vi "Write Record.vi"(8 "error in (no error)":errorcluster, 10 "Record":T1 {"Balance" format="%_4p"}, 11 "Simulated Configuration Database Actor in":refnum<class "Configuration Database Actor.lvclass">) -> (0 "error out":errorcluster, 3 "Simulated Configuration Database Actor out":refnum<class "Configuration Database Actor.lvclass">)   [LabVIEW 2019, in "Configuration Database Actor.lvlib" / "Configuration Database Actor.lvclass"]
uses:
  Configuration Database Actor.lvclass
  Records -cluster.ctl
  Configuration Database Actor.lvclass/Configuration Database Actor.ctl
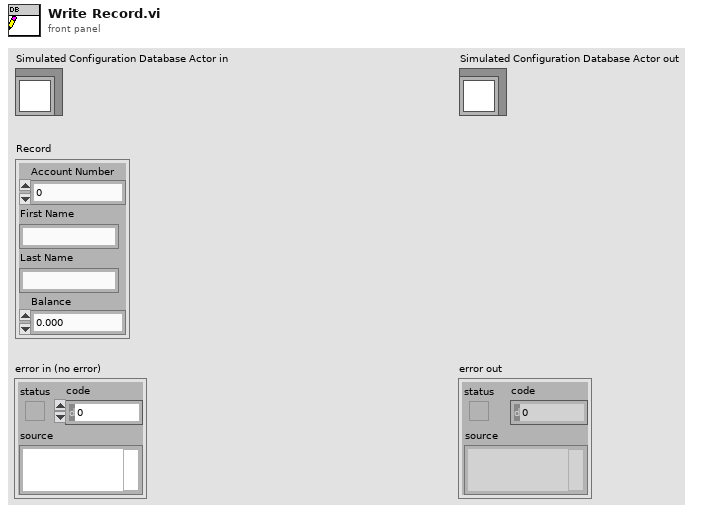
[diagram p1: front panel]
types:
  T1 = typedef "Configuration Database Actor.lvlib/Configuration Database Actor.lvclass/Records -cluster.ctl" = cluster{"Account Number":i32, "First Name":string, "Last Name":string, "Balance":i32}
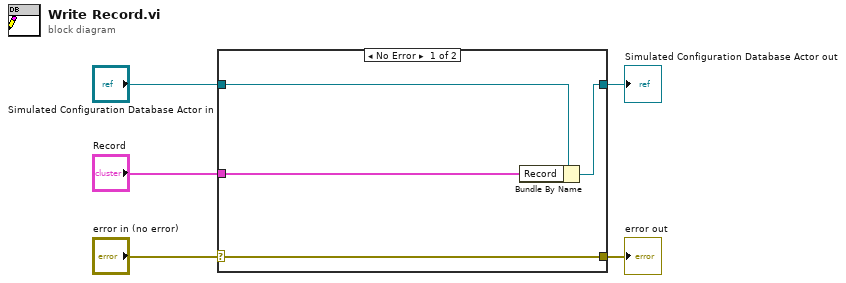
[diagram p0: block diagram]
diagram:
  n1 = case shown="No Error" "error in (no error)" {
    selector: "error in (no error)" -> [w9 w10]
    tunnel: [w9 w10] -> w4
    tunnel: [w7 w11] -> w2
    tunnel: "Simulated Configuration Database Actor in" -> [w8 w11]
    tunnel: "Record" -> [w6 _]
    frame No Error {
      n2 = Bundle By Name(cluster=w8, "Record"=w6) -> (w7:refnum<class "Configuration Database Actor.lvclass">)
    }
    frame Error {
    }
  }
  "error out" <- w4
  "Simulated Configuration Database Actor out" <- w2
